vi "Rec2Pol9225-7_FPGA.vi"(2 "Imag":fxp<+/-,36,0>, 3 "Real":fxp<+/-,36,0>) -> (0 "phase [pi]":fxp<+/-,36,2>, 1 "magnitude [p.u.]":fxp<+,36,0>)   [LabVIEW 2021]
uses:
  <vilib>/rvi/FXPMathLib/FxpRectToPolar/subVIs/nifxpmath_RectToPolar_SimConfig.ctl
  <vilib>/rvi/FXPMathLib/FxpRectToPolar/simVIs/DllFxpRectToPolarTemp_sub.vi
  <vilib>/rvi/FXPMathLib/FxpRectToPolar/XNode/nifxpmath_RectToPolar.xnode
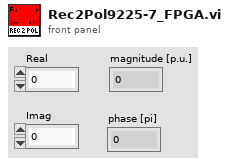
[diagram p1: front panel]
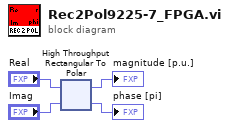
[diagram p0: block diagram]
diagram:
  n1 = xnode "High Throughput Rectangular To Polar"("x"="Real", "y"="Imag") -> ("magnitude"=→"magnitude [p.u.]":fxp<+,36,0>, "phase (pi)"=→"phase [pi]":fxp<+/-,36,2>)
